vi "KVMap-From String.vi"(11 "value":string) -> (3 "Cluster":cluster{string[], string[]})   [LabVIEW 2014]
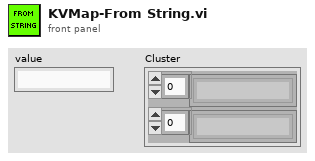
[diagram p1: front panel]
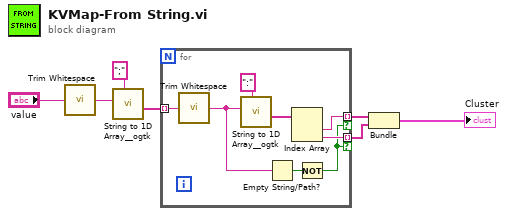
[diagram p0: block diagram]
diagram:
  n1 = call <vilib>:"Trim Whitespace.vi"("string"="value") -> ("trimmed string"=w4:string)  [unwired: 1 in]
  n2 = call <userlib>:"String to 1D Array__ogtk.vi"("delimiter (Tab)"=";", "string"=w4) -> ("Array of Strings"=w3:string[])  [unwired: 9 in]
  n3 = for {
    tunnel: w3 -> [w11] mode=indexing
    tunnel: [w13] -> w5 mode=indexing if=w8
    tunnel: [w12] -> w6 mode=indexing if=w8
    n4 = call <vilib>:"Trim Whitespace.vi"("string"=w11) -> ("trimmed string"=w10:string)  [unwired: 1 in]
    n5 = call <userlib>:"String to 1D Array__ogtk.vi"("delimiter (Tab)"=":", "string"=w10) -> ("Array of Strings"=w14:string[])  [unwired: 9 in]
    n6 = Empty String/Path?(string/path=w10) -> (empty?=w9:bool)
    n7 = Index Array(array=w14) -> (element #1=w13:string, element #2=w12:string)  [unwired: 2 in]
    n8 = Not(x=w9) -> (.not. x?=w8:bool)
  }
  n9 = Bundle(w5, w6) -> (→"Cluster":cluster{string[], string[]})  [unwired: 1 in]
